vi "PID.vi"(0 "Kp":dbl, 1 "Process Variable":dbl, 2 "Goal":dbl, 5 "Ki":dbl, 7 "Kd":dbl, 9 "N-Diff":i32=3, 11 "N-Int":i32=12, 12 "Reinit":bool, 13 "Max Ouput":dbl=1.0, 14 "Min Output":dbl=-1.0) -> (4 "Current Error":dbl, 8 "Command":dbl, 15 "PID Tracking":cluster{"Goal Wheel Position":dbl, dbl}(graph)={"Goal Wheel Position"=0.0, -90.17571233858979})   [LabVIEW 2019]
uses:
  <vilib>/Analysis/NI_AALPro.lvlib
panel:
  out "Absolute Iterations":i32
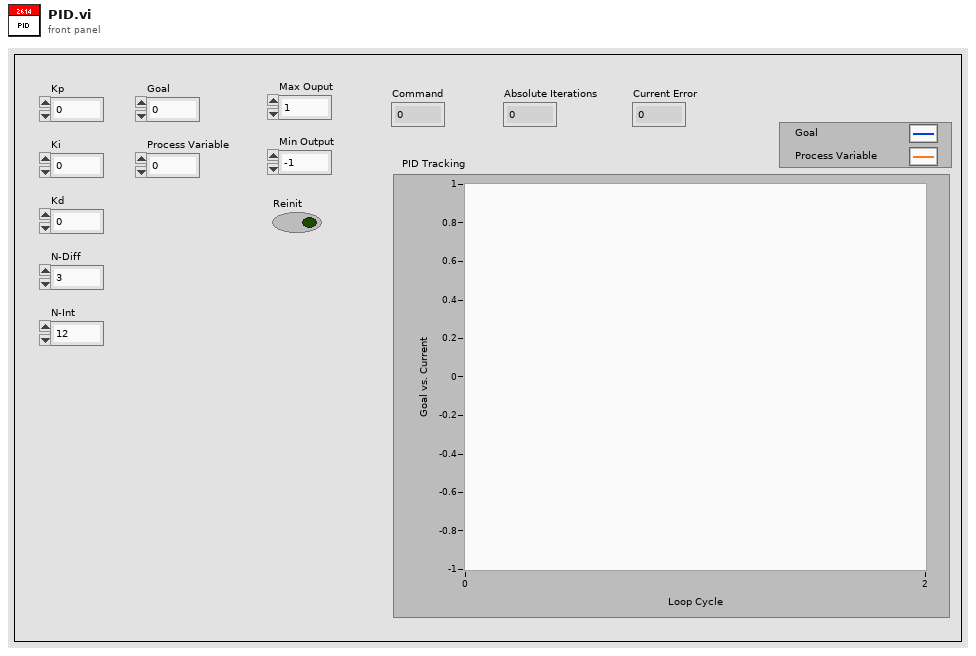
[diagram p1: front panel]
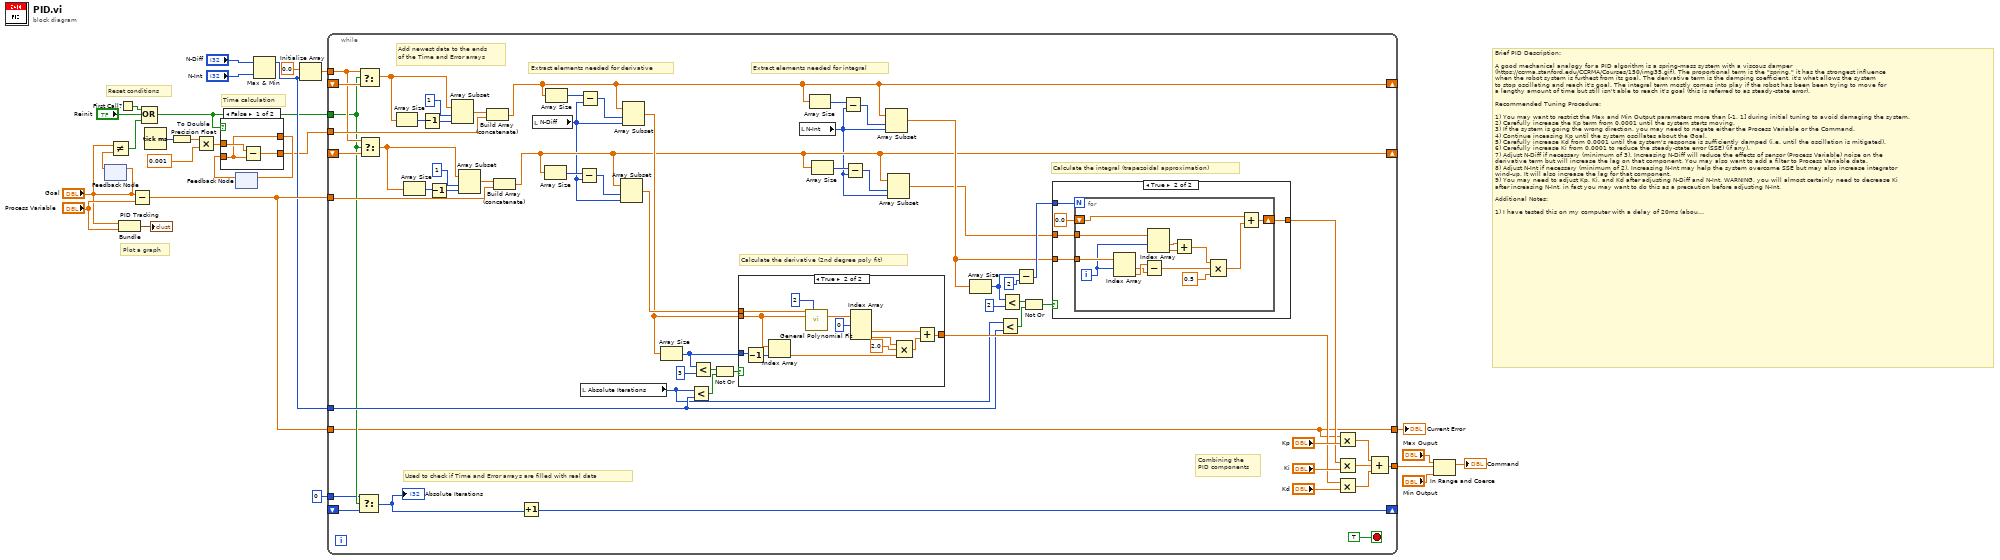
[diagram p0: block diagram]
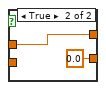
[diagram p2: hidden frame]
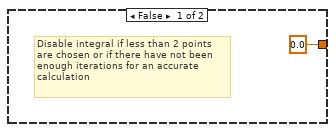
[diagram p3: hidden frame]
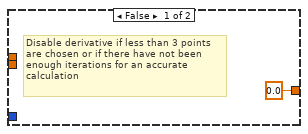
[diagram p4: hidden frame]
diagram:
  # "Time calculation"
  # "Brief PID Description:\n\nA good mechanical analogy for a PID algorithm is a spring-mass system with a viscous damper \n(https://ccrma.stanford.edu/CCRMA/Courses/150/img35.gif). The proportional term is the \"spring,\" it has the strongest influence\nwhen the robot system is furthest from its goal. The derivative term is the damping coefficient, it's what allows the system\nto stop oscillating and reach it's goal. The integral term mostly comes into play if the robot has been been trying to move for \na lengthy amount of time but still isn't able to reach it's goal (this is referred to as steady-state error).\n\nRecommended Tuning Procedure:\n\n1) You may want to restrict the Max and Min Output parameters more than [-1, 1] during initial tuning to avoid damaging the system.\n2) Carefully increase the Kp term from 0.0001 until the system starts moving.\n3) If the system is going the wrong direction, you may need to negate either the Process Variable or the Command.\n4) Continue inceasing Kp until the system oscillates about the Goal.\n5) Carefully increase Kd from 0.0001 until the system's response is sufficiently damped (i.e. until the oscillation is mitigated).\n6) Carefully increase Ki from 0.0001 to reduce the steady-state error (SSE) (if any).\n7) Adjust N-Diff if necessary (minimum of 3). Increasing N-Diff will reduce the effects of sensor (Process Variable) noise on the \nderivative term but will increase the lag on that component. You may also want to add a filter to Process Variable data.\n8) Adjust N-Int if necessary (minimum of 2). Increasing N-Int may help the system overcome SSE but may also increase integrator\nwind-up. It will also increase the lag for that component.\n9) You may need to adjust Kp, Ki, and Kd after adjusting N-Diff and N-Int. WARNING, you will almost certainly need to decrease Ki\nafter increasing N-Int, in fact you may want to do this as a precaution before adjusting N-Int. \n\nAdditional Notes:\n\n1) I have tested this on my computer with a delay of 20ms (about what I expect for the robot) and it appears to function correctly.\nThat being said I have NOT tested this on an actual, physical system. So exercise caution when testing it for the first time.\n2) Make sure that execution type for all instances of this VI are set to \"preallocated clone reentrant execution.\"\n3) Several parts of this VI were inspired by a PID algorithm written by Dr. Ira Hill at the University of Florida.\n4) If you have any questions, feel free to contact me at lrscime@ufl.edu."
  # "Plot a graph"
  # "Reset conditions"
  n1 = feedback-in #1("Goal") -> ()
  n2 = feedback #1() -> (w12:dbl)  [unwired: 1 in]
  n3 = Not Equal?(x="Goal", y=w12) -> (x != y?=w11:bool)
  n4 = First Call?() -> (First Call?: T/F=w20:bool)
  n5 = Bundle("Goal"="Goal", "Process Variable"="Process Variable") -> (→"PID Tracking":cluster{"Goal":dbl, "Process Variable":dbl})  [unwired: 1 in]
  n6 = Subtract(x="Goal", y="Process Variable") -> (x-y=w27:dbl)
  n7 = Compound Arithmetic op=OR(w20, "Reinit", w11) -> (w2:bool)
  n8 = Tick Count (ms)() -> (millisecond timer value=w9:u32)
  n9 = To Double Precision Float(number=w9) -> (double precision float=w8:dbl)
  n10 = Multiply(x=w8, y=0.001) -> (x*y=w6:dbl)
  n11 = feedback #2() -> (w4:dbl)  [unwired: 1 in]
  n12 = case shown="False" w2 {
    tunnel: w6 -> [w30 w32]
    tunnel: [w28 w32] -> w5
    tunnel: [w29 0.0] -> w3
    tunnel: w4 -> [w28 _]
    frame False {
      n13 = Subtract(x=w30, y=w28) -> (x-y=w29:dbl)
    }
    frame True {
    }
  }
  n14 = feedback-in #2(w5) -> ()
  n15 = Max & Min(x="N-Diff", y="N-Int") -> (max(x,y)=w14:i32)  [unwired: 1 out]
  n16 = Initialize Array(0.0 ("element"), w14) -> (w16:dbl[])
  n17 = while {
    tunnel: [w86] -> w24
    tunnel: w27 -> [w77]
    shift-right: [w61] -> _
    shift-left: _ -> [w46]
    tunnel: w3 -> [w81]
    shift-right: [w47] -> _
    shift-left: _ -> [w43]
    tunnel: w14 -> [w53]
    tunnel: w27 -> [w33]
    shift-right: [w54] -> _
    shift-left: _ -> [w40]
    tunnel: w2 -> [w39]
    tunnel: w16 -> [w44]
    tunnel: 0 -> [w35]
    tunnel: [w33] -> w1
    stop <- TRUE stop-if-true
    # "Combining the\nPID components"
    # "Add newest data to the ends\nof the Time and Error arrays"
    # "Used to check if Time and Error arrays are filled with real data"
    # "Extract elements needed for integral"
    # "Extract elements needed for derivative"
    # "Calculate the integral (trapezoidal approximation)"
    # "Calculate the derivative (2nd degree poly fit)"
    n18 = Select(t=w35, s=w39, f=w40) -> (s? t:f=w41:i32)
    "Absolute Iterations" <- w41
    n19 = Select(t=w44, s=w39, f=w46) -> (s? t:f=w45:dbl[])
    n20 = Select(t=w44, s=w39, f=w43) -> (s? t:f=w42:dbl[])
    n21 = Array Size(array=w45) -> (size(s)=w84:i32)
    n22 = Array Size(array=w42) -> (size(s)=w79:i32)
    n23 = Decrement(x=w84) -> (x-1=w83:i32)
    n24 = Decrement(x=w79) -> (x-1=w78:i32)
    n25 = Array Subset(array=w45, index=1, length=w83) -> (w82:dbl[])
    n26 = Array Subset(array=w42, index=1, length=w78) -> (w76:dbl[])
    n27 = Build Array (concatenate)(w82, w81) -> (w61:dbl[])
    n28 = Build Array (concatenate)(w76, w77) -> (w47:dbl[])
    n29 = Increment(x=w41) -> (x+1=w54:i32)
    n30 = local read "N-Diff"() -> (w37:i32)
    n31 = Array Size(array=w47) -> (size(s)=w72:i32)
    n32 = Array Size(array=w61) -> (size(s)=w75:i32)
    n33 = Subtract(x=w72, y=w37) -> (x-y=w73:i32)
    n34 = Subtract(x=w75, y=w37) -> (x-y=w74:i32)
    n35 = local read "Absolute Iterations"() -> (w34:i32)
    n36 = Array Subset(array=w47, index=w73, length=w37) -> (w71:dbl[])
    n37 = Array Subset(array=w61, index=w74, length=w37) -> (w70:dbl[])
    n38 = Array Size(array=w70) -> (size(s)=w68:i32)
    n39 = Less?(x=w34, y=w53) -> (x < y?=w66:bool)
    n40 = Less?(x=w68, y=3) -> (x < y?=w69:bool)
    n41 = Not Or(1:w66, 2:w69) -> (0:w65:bool)
    n42 = case shown="True" w65 {
      tunnel: w71 -> [_ w119]
      tunnel: w68 -> [_ w118]
      tunnel: w70 -> [_ w116]
      tunnel: [0.0 w114] -> w64
      frame False {
        # "Disable derivative if less than 3 points \nare chosen or if there have not been \nenough iterations for an accurate \ncalculation"
      }
      frame True {
        n43 = Decrement(x=w118) -> (x-1=w117:i32)
        n44 = Index Array(array=w116, index=w117) -> (element=w115:dbl)
        n45 = call <vilib>:"General Polynomial Fit.vi"("Y"=w119, "polynomial order"=2, "X"=w116) -> ("Polynomial Coefficients"=w125:dbl[])  [unwired: 9 in, 3 out]
        n46 = Index Array(array=w125, index #1=0 ("index")) -> (element #2=w121:dbl, element #3=w123:dbl)  [unwired: 2 in, 1 out]
        n47 = Compound Arithmetic op=MULTIPLY(w123, 2.0 ("y"), w115) -> (w120:dbl)
        n48 = Add(x=w121, y=w120) -> (x+y=w114:dbl)
      }
    }
    n49 = local read "N-Int"() -> (w36:i32)
    n50 = Array Size(array=w61) -> (size(s)=w63:i32)
    n51 = Array Size(array=w47) -> (size(s)=w60:i32)
    n52 = Subtract(x=w63, y=w36) -> (x-y=w62:i32)
    n53 = Subtract(x=w60, y=w36) -> (x-y=w59:i32)
    n54 = Array Subset(array=w61, index=w62, length=w36) -> (w48:dbl[])
    n55 = Array Subset(array=w47, index=w59, length=w36) -> (w38:dbl[])
    n56 = Array Size(array=w48) -> (size(s)=w51:i32)
    n57 = Less?(x=w34, y=w53) -> (x < y?=w56:bool)
    n58 = Less?(x=w51, y=2) -> (x < y?=w58:bool)
    n59 = Subtract(x=w51, y=2) -> (x-y=w50:i32)
    n60 = Not Or(1:w56, 2:w58) -> (0:w55:bool)
    n61 = case shown="True" w55 {
      tunnel: [0.0 w97] -> w52
      tunnel: w50 -> [_ w99]
      tunnel: w48 -> [_ w96]
      tunnel: w38 -> [_ w95]
      frame False {
        # "Disable integral if less than 2 points \nare chosen or if there have not been \nenough iterations for an accurate \ncalculation"
      }
      frame True {
        n62 = for {
          N: w99 -> [_]
          shift-right: [w111] -> w97
          shift-left: 0.0 -> [w112]
          tunnel: w96 -> [w110]
          tunnel: w95 -> [w103]
          i -> [w104]
          n63 = Index Array(array=w110, index #1=w104) -> (element #1=w108:dbl, element #2=w109:dbl)  [unwired: 1 in]
          n64 = Subtract(x=w109, y=w108) -> (x-y=w107:dbl)
          n65 = Index Array(array=w103, index #1=w104) -> (element #1=w101:dbl, element #2=w102:dbl)  [unwired: 1 in]
          n66 = Add(x=w101, y=w102) -> (x+y=w100:dbl)
          n67 = Compound Arithmetic op=MULTIPLY(w100, w107, 0.5 ("value")) -> (w105:dbl)
          n68 = Add(x=w112, y=w105) -> (x+y=w111:dbl)
        }
      }
    }
    n69 = Multiply(x=w33, y="Kp") -> (x*y=w93:dbl)
    n70 = Multiply(x=w52, y="Ki") -> (x*y=w92:dbl)
    n71 = Multiply(x=w64, y="Kd") -> (x*y=w91:dbl)
    n72 = Compound Arithmetic op=ADD(w93, w92, w91) -> (w86:dbl)
  }
  "Current Error" <- w1
  n73 = In Range and Coerce(upper limit="Max Ouput", x=w24, lower limit="Min Output") -> (coerced(x)=→"Command":dbl)  [unwired: 1 out]
